vi "CheckConnection.vi"(8 "error in (no error)":errorcluster, 9 "Blocking?":bool, 10 "Timeout (5000 ms)":i32=5000, 11 "BASE.Device in":refnum<class "BASE.Device.lvclass">) -> (0 "error out":errorcluster, 3 "BASE.Device out":refnum<class "BASE.Device.lvclass">)   [LabVIEW 2019, in "BASE.Device.lvlib" / "BASE.Device.lvclass"]
uses:
  BASE.Device.lvclass
  D:/Program Files (x86)/National Instruments/LabVIEW 2019/vi.lib/ActorFramework/Actor/Actor.lvclass
  BASE.Device.lvclass/BASE.Device.ctl
  <vilib>/ActorFramework/Actor/Actor.lvclass/Actor.ctl
  <vilib>/ActorFramework/Message Enqueuer/Message Enqueuer.lvclass/Message Enqueuer.ctl
  BASE.Device Messages/CheckConnection Msg/CheckConnection Msg.lvclass/CheckConnection Msg.ctl
  <vilib>/ActorFramework/Message Enqueuer/Init from Existing Queue.vi
  <vilib>/ActorFramework/Message Enqueuer/Enqueue.vi
  BASE.Device Messages/CheckConnection Msg/CheckConnection Msg.lvclass
  D:/Program Files (x86)/National Instruments/LabVIEW 2019/vi.lib/ActorFramework/Message/Message.lvclass
  <vilib>/ActorFramework/Message Priority Queue/Priority Enqueue.vi
  <vilib>/ActorFramework/Message Enqueuer/Message Enqueuer.lvclass
  <vilib>/ActorFramework/Actor/Actor.lvclass
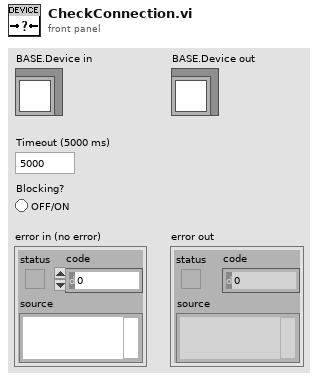
[diagram p1: front panel]
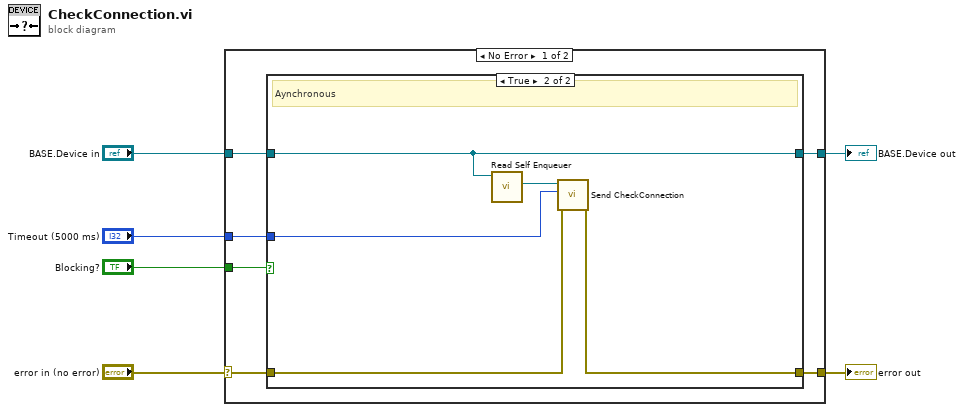
[diagram p0: block diagram]
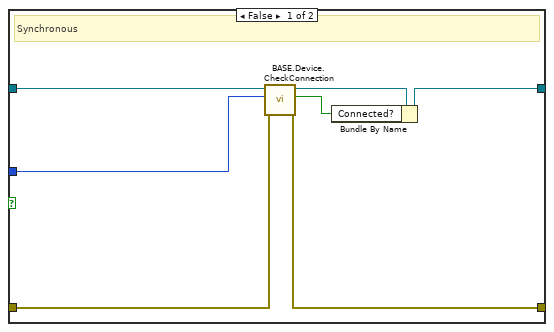
[diagram p2: hidden frame]
diagram:
  n1 = case shown="No Error" "error in (no error)" {
    selector: "error in (no error)" -> [w9 w26]
    tunnel: [w8 w26] -> w5
    tunnel: [w10 w25] -> w3
    tunnel: "BASE.Device in" -> [w11 w25]
    tunnel: "Timeout (5000 ms)" -> [w12 _]
    tunnel: "Blocking?" -> [w7 _]
    frame No Error {
      n2 = case shown="True" w7 {
        tunnel: w12 -> [w19 w24]
        tunnel: w11 -> [w18 w21]
        tunnel: [w14 w21] -> w10
        tunnel: w9 -> [w17 w23]
        tunnel: [w16 w22] -> w8
        frame False {
          # "Synchronous"
          n3 = call-dynamic "BASE.Device.CheckConnection.vi"("error in (no error)"=w17, "Timeout (5000 ms)"=w19, "BASE.Device in"=w18) -> ("error out"=w16:errorcluster, "Connected?"=w13:bool, "BASE.Device out"=w15:refnum<class "BASE.Device.lvclass">)  [unwired: 6 in]
          n4 = Bundle By Name(cluster=w15, "Connected?"=w13) -> (w14:refnum<class "BASE.Device.lvclass">)
        }
        frame True {
          # "Aynchronous"
          n5 = call <vilib>:"Read Self Enqueuer.vi"("Actor"=w21) -> ("Self Enqueuer"=w20:refnum<class "Message Enqueuer.lvclass">)  [unwired: 10 in]
          n6 = call "Send CheckConnection.vi"("error in (no error)"=w23, "Timeout (5000 ms)"=w24, "Message Enqueuer"=w20) -> ("error out"=w22:errorcluster)  [unwired: 7 in, 1 out]
        }
      }
    }
    frame Error {
    }
  }
  "error out" <- w5
  "BASE.Device out" <- w3
